vi "setUp.vi"(8 "error in (no error)":errorcluster, 11 "reference in":refnum<class "testcase-csm-file-logger.lvclass">) -> (0 "error out":errorcluster, 3 "reference out":refnum<class "testcase-csm-file-logger.lvclass">)   [LabVIEW 2017, in "testcase-csm-file-logger.lvclass"]
doc: "setUp runs prior to the test method during test execution. Use this method to initialize any object data required by your tests."
uses:
  testcase-csm-file-logger.lvclass
  C:/Program Files (x86)/National Instruments/LabVIEW 2017/vi.lib/addons/_JKI Toolkits/VI Tester/TestCase.llb/TestCase.lvclass
  testcase-csm-file-logger.lvclass/testcase-csm-file-logger.ctl
  <vilib>/addons/_JKI Toolkits/VI Tester/TestCase.llb/TestCase.lvclass
  src/examples/NEVSTOP/Communicable State Machine(CSM)/1. Create a reuse Module/1. Create a reuse Module.lvlib
  src/user.lib/_NEVSTOP/Communicable State Machine(CSM)/Communicable State Machine.lvlib
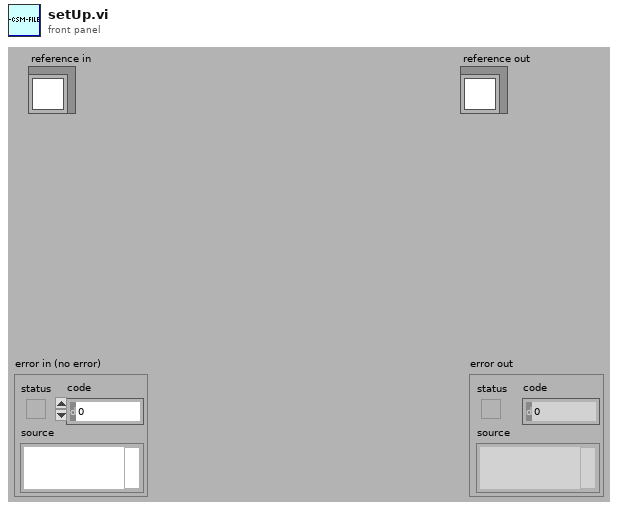
[diagram p1: front panel]
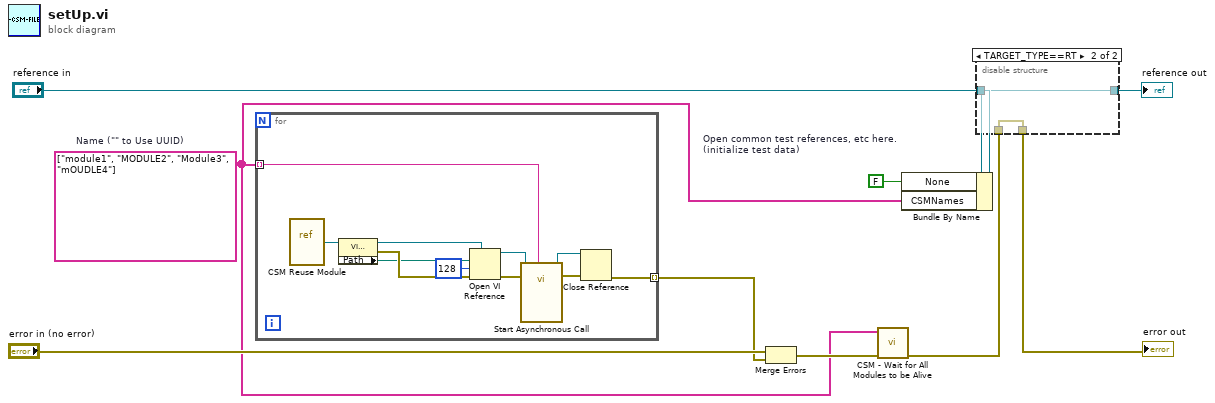
[diagram p0: block diagram]
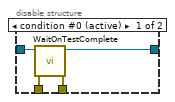
[diagram p2: hidden frame]
diagram:
  w1 = string[] ["module1", "MODULE2", "Module3", "mOUDLE4"]  # Name ("" to Use UUID)
  w5 = FALSE  # Open common test references, etc here. (initialize test data)
  n1 = for {
    tunnel: w1 -> [w18] mode=indexing
    tunnel: [w11] -> w3 mode=indexing
    n2 = vi-ref "CSM Reuse Module.vi"() -> (w13:refnum<vi>)
    n3 = property class="VI (strict)"(reference=w13) -> (reference out=w17:refnum<vi>, error out=w15:errorcluster, "Path"=w14:path)  [unwired: 1 in]
    n4 = Open VI Reference(type specifier VI Refnum (for type only)=w17, vi path=w14, options=128, error in (no error)=w15) -> (vi reference=w16:refnum<vi>, error out=w12:errorcluster)  [unwired: 2 in]
    n5 = call-by-ref "Start Asynchronous Call"(reference=w16, error in=w12, "Name(\"\" to use uuid)"=w18) -> (reference out=w20:refnum<vi>, error out=w19:errorcluster)  [unwired: 11 in]
    n6 = Close Reference(reference=w20, error in (no error)=w19) -> (error out=w11:errorcluster)
  }
  n7 = Merge Errors("error in (no error)", w3) -> (w4:errorcluster)
  n8 = call "CSM - Wait for All Modules to be Alive.vi"("Error In"=w4, "CSM Names"=w1) -> ("error out"=w2:errorcluster)  [unwired: 7 in, 2 out]
  n9 = Bundle By Name(cluster="reference in", "None"=w5, "CSMNames"=w1) -> (w6:refnum<class "testcase-csm-file-logger.lvclass">)
  n10 = disable-structure shown="TARGET_TYPE==RT" {
    disable-tunnel: w2 -> [w25 w26]
    disable-tunnel: [w24 w26] -> w9
    disable-tunnel: [w23 w27] -> w7
    disable-tunnel: w6 -> [w22 w27]
    frame condition #0 (active) {
      n11 = call <vilib>:"WaitOnTestComplete.vi"("error in (no error)"=w25, "TestCase in"=w22) -> ("error out"=w24:errorcluster, "TestCase out"=w23:refnum<class "testcase-csm-file-logger.lvclass">)  [unwired: 8 in]
    }
    frame condition #1 {
    }
  }
  "error out" <- w9
  "reference out" <- w7
